vi "工具_随机密码生成.vi"(7 "长度":u32=48, 8 "布尔_特殊字符":bool, 9 "布尔_大写字母":bool=TRUE, 10 "布尔_小写字母":bool=TRUE, 11 "布尔_数字":bool=TRUE) -> (3 "随机密码":string)   [LabVIEW 2014]
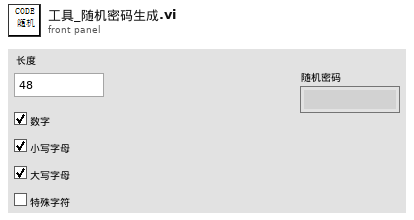
[diagram p1: front panel]
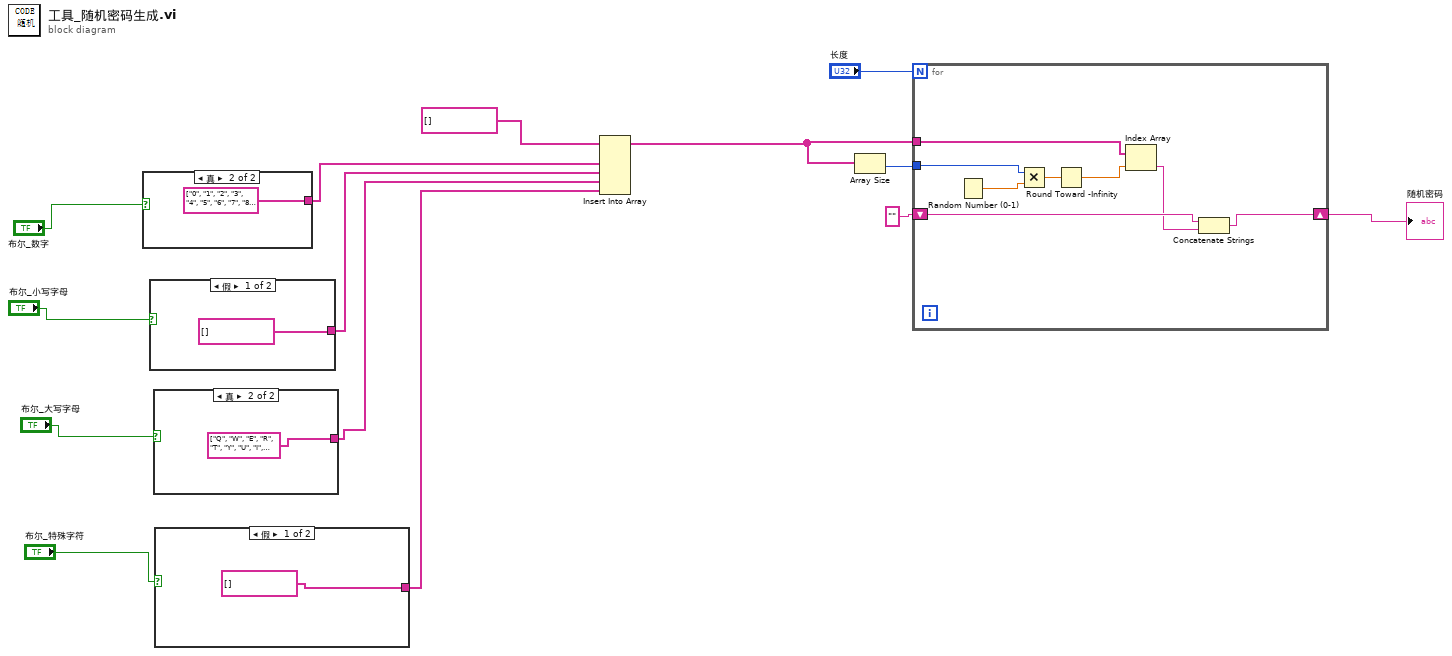
[diagram p0: block diagram]
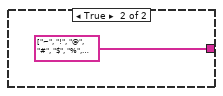
[diagram p2: hidden frame]
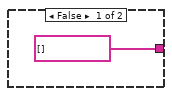
[diagram p3: hidden frame]
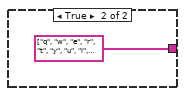
[diagram p4: hidden frame]
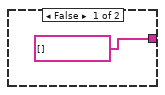
[diagram p5: hidden frame]
diagram:
  n1 = case shown="真" "布尔_数字" {
    tunnel: [string[] [] string[] ["0", "1", "2", "3", "4", "5", "6", "7", "8", "9"]] -> w9
    frame False {
    }
    frame True {
    }
  }
  n2 = case shown="假" "布尔_小写字母" {
    tunnel: [string[] [] string[] ["q", "w", "e", "r", "t", "y", "u", "i", "o", "p", "a", "s", "d", "f", "g", "h", "j", "k", "l", "z", "x", "c", "v", "b", "n", "m"]] -> w8
    frame False {
    }
    frame True {
    }
  }
  n3 = case shown="真" "布尔_大写字母" {
    tunnel: [string[] [] string[] ["Q", "W", "E", "R", "T", "Y", "U", "I", "O", "P", "A", "S", "D", "F", "G", "H", "J", "K", "L", "Z", "X", "C", "V", "B", "N", "M"]] -> w7
    frame False {
    }
    frame True {
    }
  }
  n4 = case shown="假" "布尔_特殊字符" {
    tunnel: [string[] [] string[] ["~", "!", "@", "#", "$", "%", "^", "&", "*", "(", ")", "_", "+"]] -> w6
    frame False {
    }
    frame True {
    }
  }
  n5 = Insert Into Array(array=string[] [], new element #1=w9, new element #2=w8, new element #3=w7, new element #4=w6) -> (w5:string[])  [unwired: 1 in]
  n6 = Array Size(array=w5) -> (size(s)=w3:i32)
  n7 = for {
    N: "长度" -> [_]
    tunnel: w5 -> [w27]
    shift-right: [w23] -> w1
    shift-left: "" -> [w25]
    tunnel: w3 -> [w29]
    n8 = Random Number (0-1)() -> (number: 0 to 1=w30:dbl)
    n9 = Multiply(x=w29, y=w30) -> (x*y=w28:dbl)
    n10 = Round Toward -Infinity(1:w28) -> (0:w26:dbl)
    n11 = Index Array(array=w27, index=w26) -> (element=w24:string)
    n12 = Concatenate Strings(w25, w24) -> (w23:string)
  }
  "随机密码" <- w1
